vi "Find Average Center.vi"(5 "Position":i32, 7 "Tray Number":i32, 9 "XYZTheta":dbl[](array[numeric]), 10 "Motion.lvclass":refnum<class "Motion.lvclass">) -> (1 "XYZTheta":dbl[](array[numeric]), 2 "Motion Out":refnum<class "Motion.lvclass">)   [LabVIEW 2016, in "Component Tray.lvclass"]
uses:
  Component Tray.lvclass
  Find Component.ctl
  Controller/Motion/Motion.lvclass
  Controller/Camera/Machine Vision.ctl
  Controller/Camera/Edmund Optics/Edmund Optics.lvclass
  D:/UCSB-Gantry/V5/Classes/Controller/Camera/Camera.lvclass
  Controller/Camera/Camera.lvclass
panel:
  in  "Speed XY":dbl=5.0
  in  "Jog Cluster":T1={"Jog XY Cluster"={"object goes up"=FALSE, "object goes down"=FALSE, "object goes right"=FALSE, "object goes left"=FALSE, "SW2"=FALSE, "SW1"=FALSE, "YY (mm)"=0.1, "YN (mm) "=0.01, "NY (mm) "=0.005, "NN (mm) "=0.001}, "Jog Z Cluster "={"Z go down 0.1 mm"=FALSE, "Z go up 0.1 mm"=FALSE, "Z go down 0.05 mm"=FALSE, "Z go up 0.05 mm"=FALSE, "Z go down 0.01 mm"=FALSE, "Z go up 0.01 mm"=FALSE, "Z go down"=FALSE, "Z go up"=FALSE, "step (mm)"=0.001}}
  in  "Go 3":bool
  in  "light":dbl=5.0
  in  "Change light":bool
  out "Image 2":T2(plugin-control)
  in  "Machine Vision 2":T3
  in  "Machine Vision":T3
  out "Gantry":dbl[](array[numeric])
  out "Sum":dbl[](array[numeric])
  out "BR XY":dbl[](array[numeric])
  out "TR XY":dbl[](array[numeric])
  out "BL XY":dbl[](array[numeric])
  out "TL XY":dbl[](array[numeric])
  in  "Record Top Right":bool
  in  "Record Bottom Right":bool
  in  "Record Bottom Left":bool
  in  "Record Top Left":bool
  in  "Go to Bottom Right":bool
  in  "Go to Top Right":bool
  in  "Go to Bottom Left":bool
  in  "Go to Top Left":bool
  in  "Joystick":bool
  out "Camera":dbl[](array[numeric])
  in  "Go to Center":bool
  in  "Component":T4
  in  "Stop Program":bool
  out "Image":T2(plugin-control)
  # "1"
  # "2"
  # "Machine Vision:\nAcrylic : None"
  # "Light \nAcrylic : 5"
  # "--> Light on  : running\n       LIght off : Finish"
  # "Position 1"
  # "Position 2"
  # "Position 3"
  # "Position 4"
  # "Acrylic PCB"
  # "3"
  # "4"
  # "5"
  # "6"
  # "7"
  # "Component alignment 定位材料"
  # "8"
  # "9"
  # "10"
  # "11"
  # "12"
  # "1. Choose pattern recognition program 選擇視覺辨識\n2. Choose camera light luminosity 選擇亮度\n3. Go To Top Left  到第一定位點，點選Joystick進行定位\n4. Record Top Left 紀錄第一點\n5. Go To Bottom Left 到第二定位點，點選Joystick進行定位\n6. Record Bottom Left 紀錄第二點\n7. Go To Top Right 到第三定位點，點選Joystick進行定位\n8. Record Bottom Left 紀錄第二點\n9. Go To Bottom Left 到第四定位點，點選Joystick進行定位\n10. Record Bottom Left 紀錄第三點\n11. Go to Center 到中心點 檢查是否定位結果正常\n12. Submit 結束Component定位"
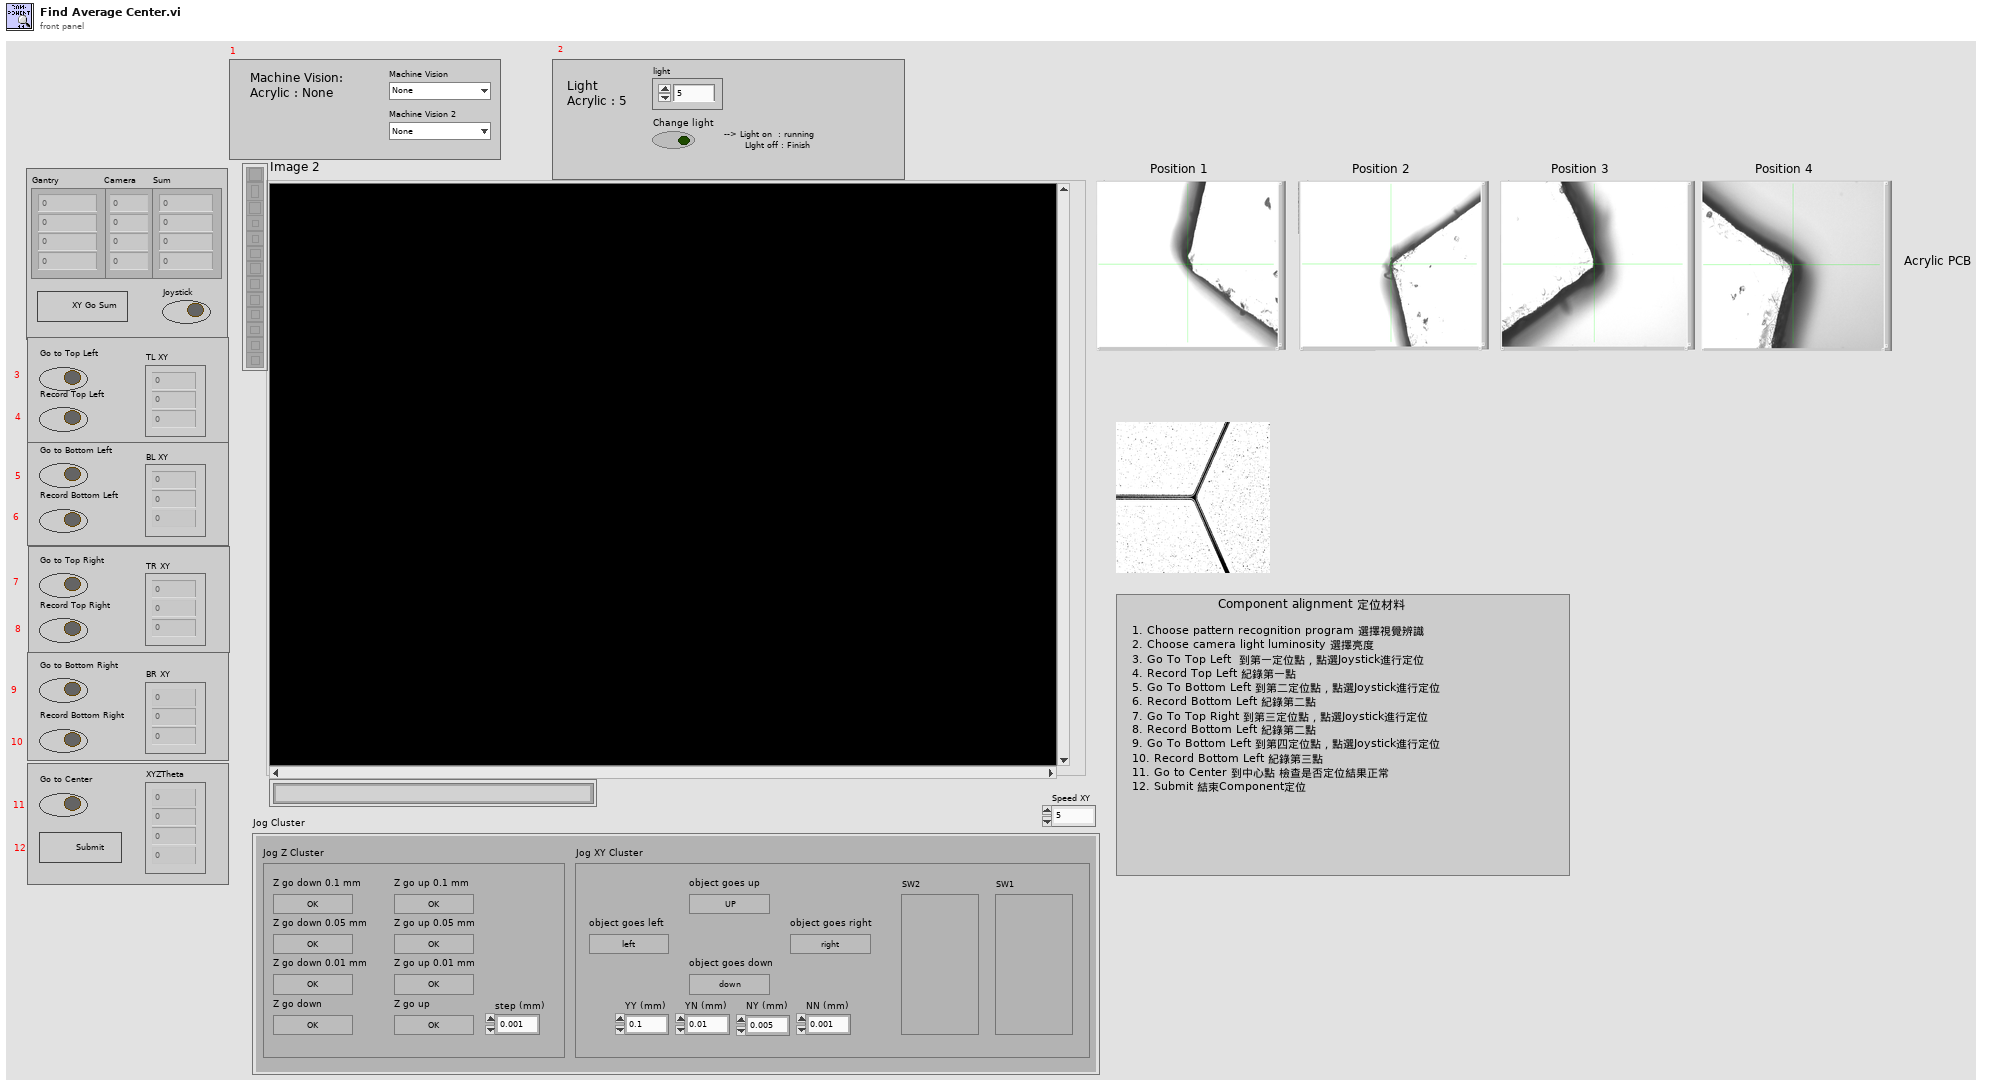
[diagram p1: front panel]
types:
  T1 = cluster{"Jog XY Cluster":cluster{"object goes up":bool, "object goes down":bool, "object goes right":bool, "object goes left":bool, "SW2":bool, "SW1":bool, "YY (mm)":dbl, "YN (mm) ":dbl, "NY (mm) ":dbl, "NN (mm) ":dbl}, "Jog Z Cluster ":cluster{"Z go down 0.1 mm":bool, "Z go up 0.1 mm":bool, "Z go down 0.05 mm":bool, "Z go up 0.05 mm":bool, "Z go down 0.01 mm":bool, "Z go up 0.01 mm":bool, "Z go down":bool, "Z go up":bool, "step (mm)":dbl}}
  T2 = typedef "IMAQ Image.ctl" = refnum<image>
  T3 = typedef "Camera.lvclass/Machine Vision.ctl" = enum16{"None", "Circle", "Tray Fiducials", "Tray Fiducials, top right", "HPK Silicon square", "HPK Silicon", "8inch PCB Pad", "Hexaboard", "Corner (TL, BR)", "Corner (BL, TR)"}
  T4 = typedef "Component Tray.lvclass/Find Component.ctl" = cluster{"New Fiducials":dbl[], "Past Fiducials":dbl[], "XYZTheta":dbl[], "Fiducials Path":path, "Position":i32}
  T5 = typedef "File Paths.ctl" = cluster{"Glue Pattern Folder":path, "Carrier Tray Folder":path, "Pick Up Tool Fixture Folder":path, "Components Folder":path, "Bellows Tool Offset.txt":path, "Pick Up Tool Offset.txt":path, "Dispense Tip Offset.txt":path, "Log Files":path}
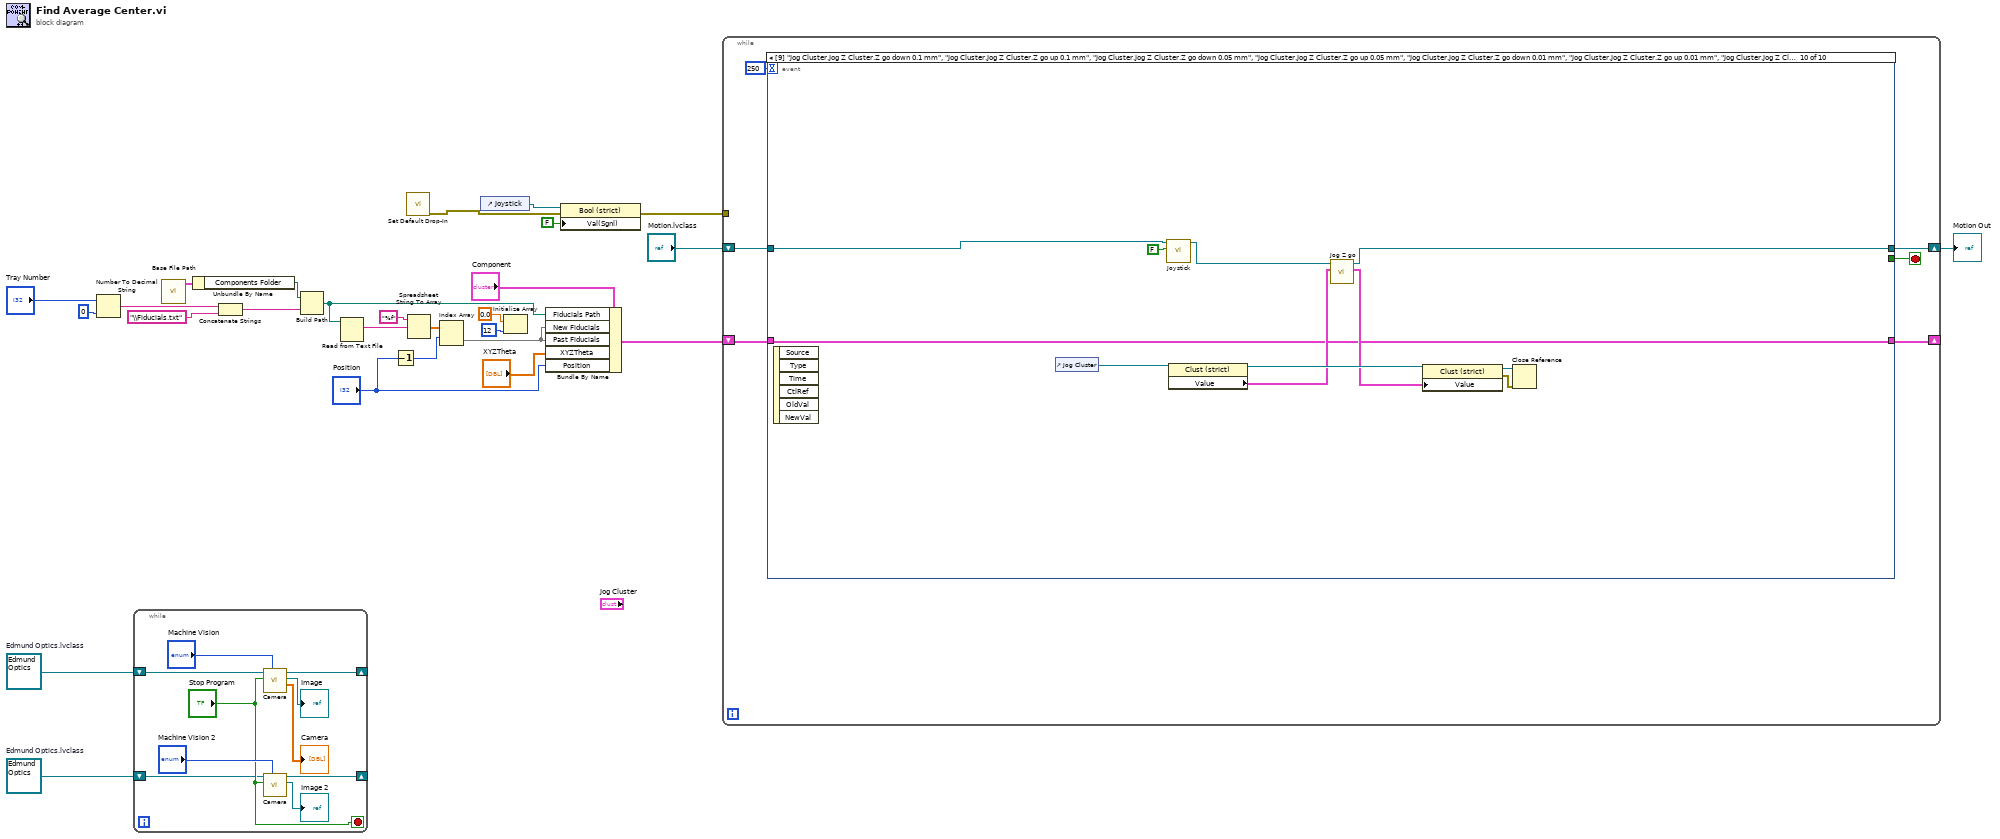
[diagram p0: block diagram]
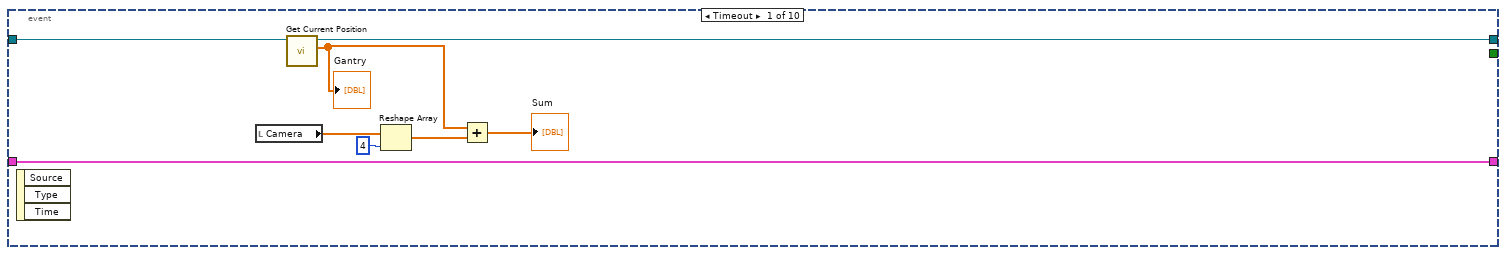
[diagram p2: hidden frame]
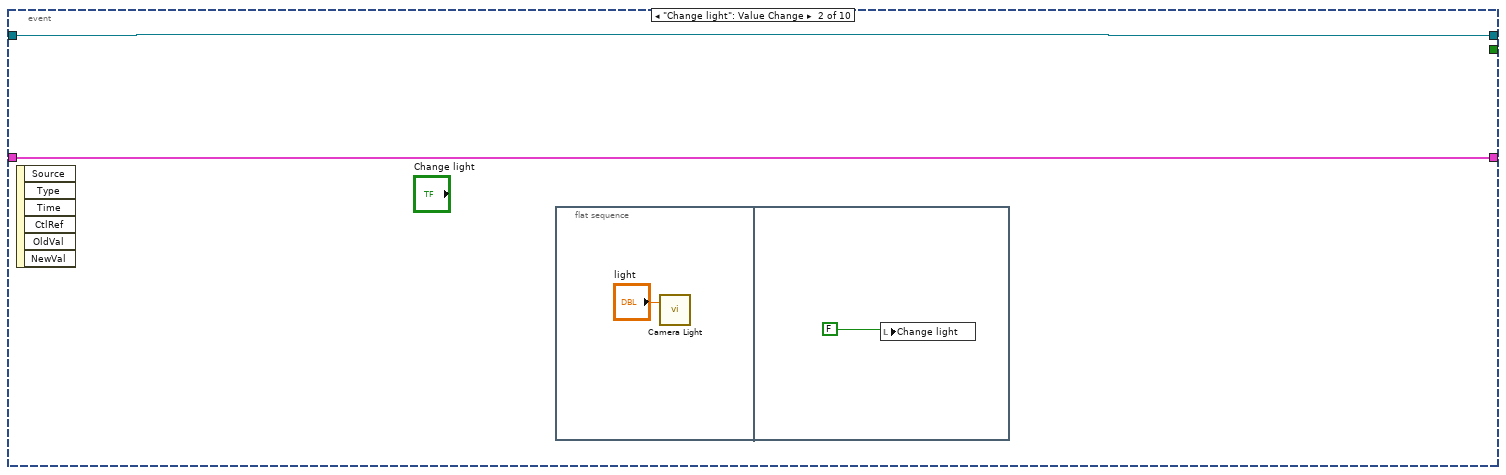
[diagram p3: hidden frame]
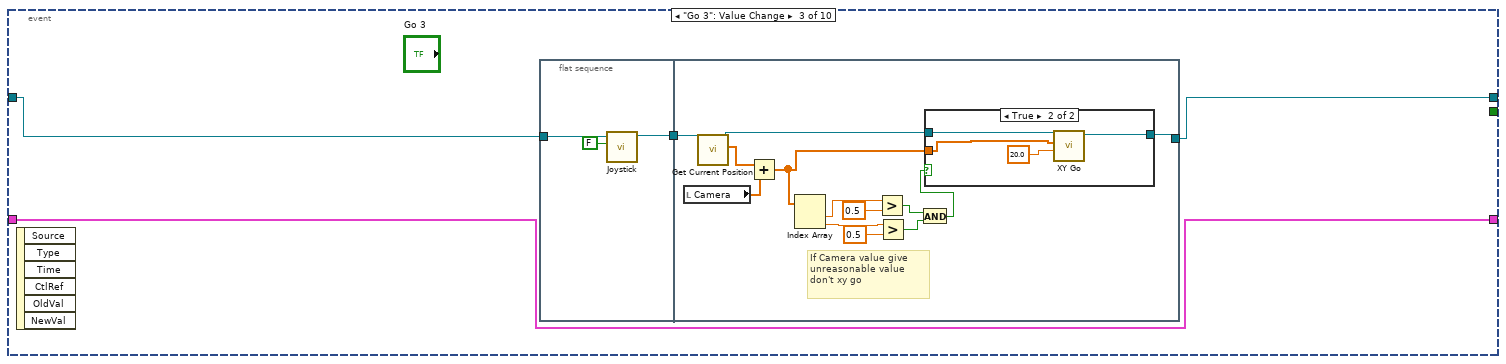
[diagram p4: hidden frame]
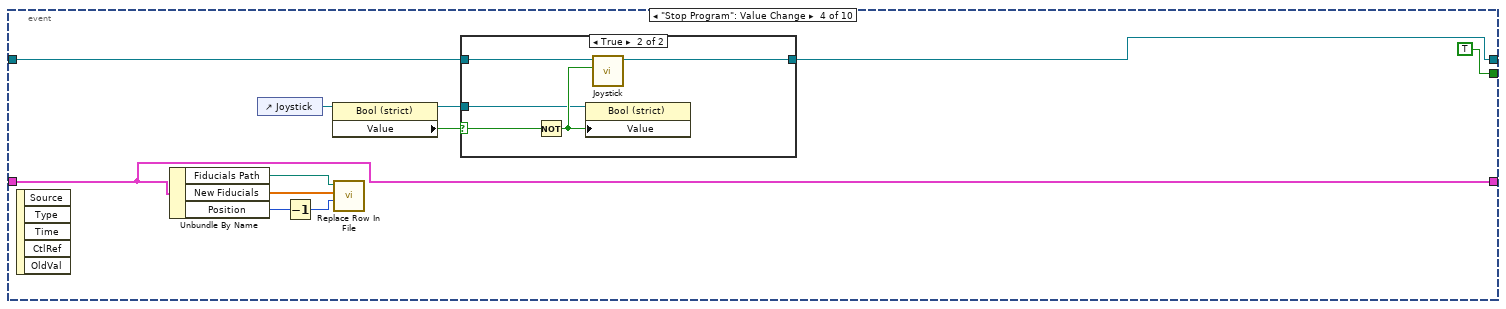
[diagram p6: hidden frame]
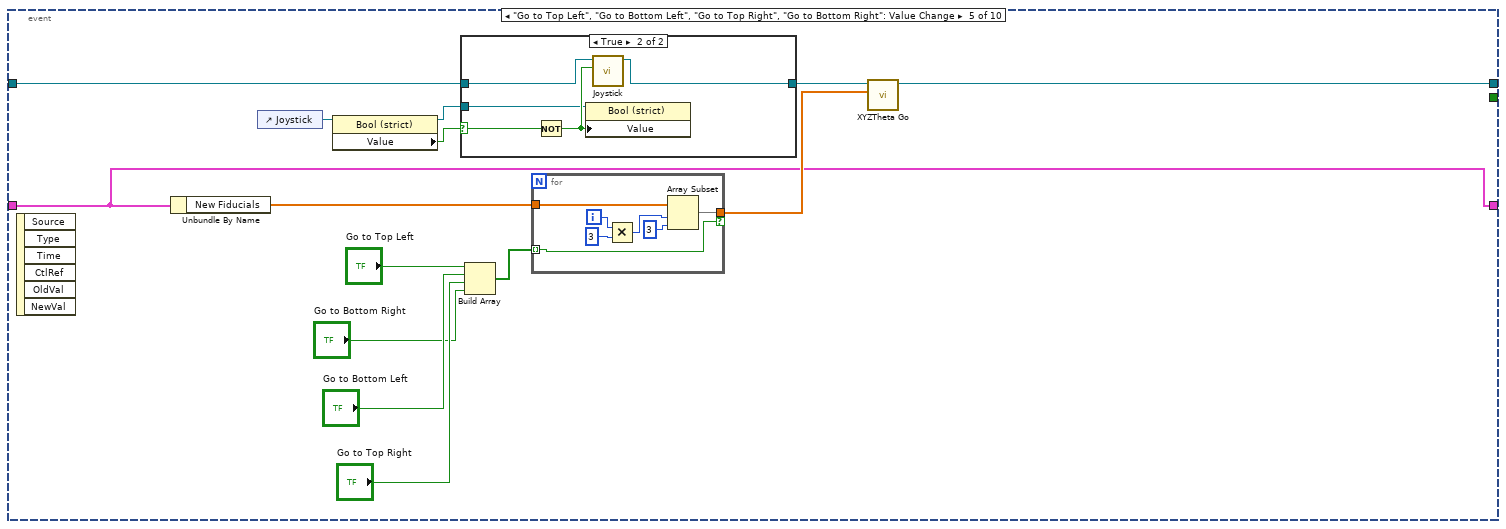
[diagram p8: hidden frame]
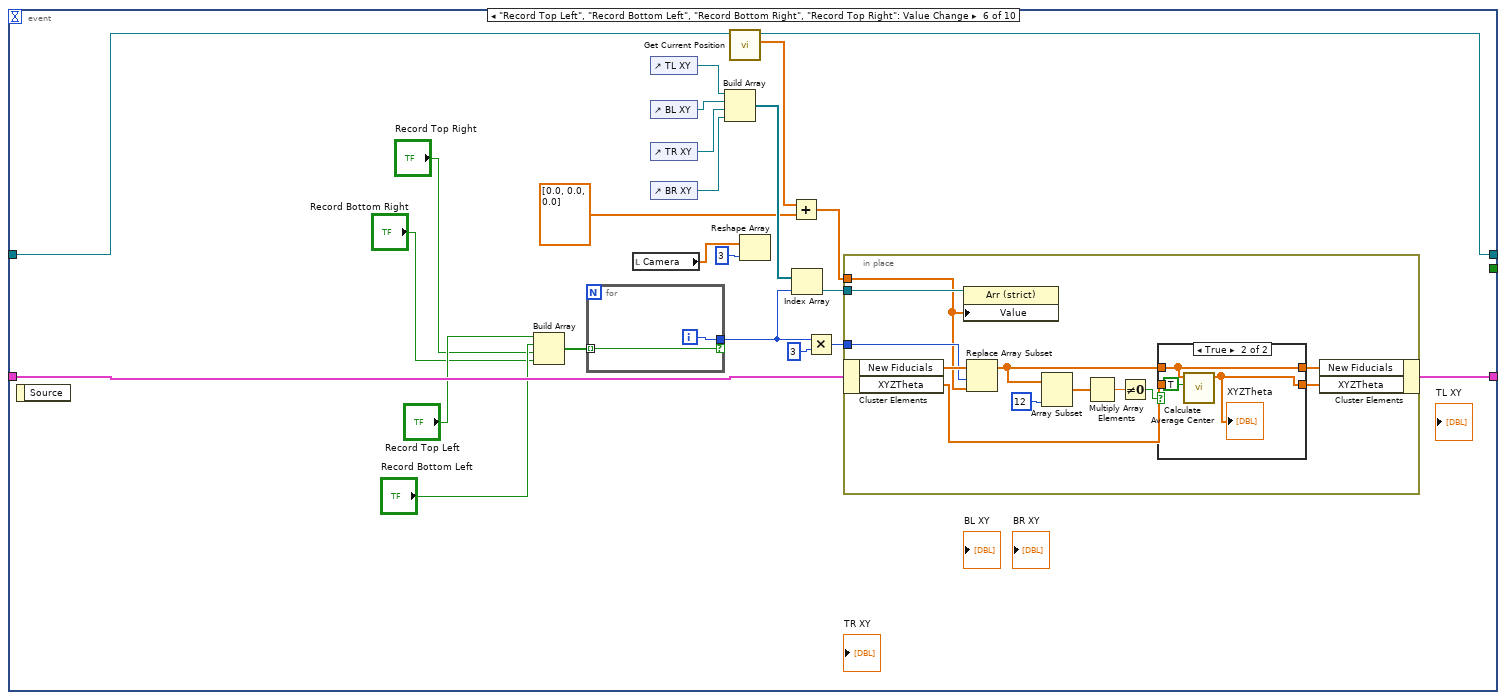
[diagram p10: hidden frame]
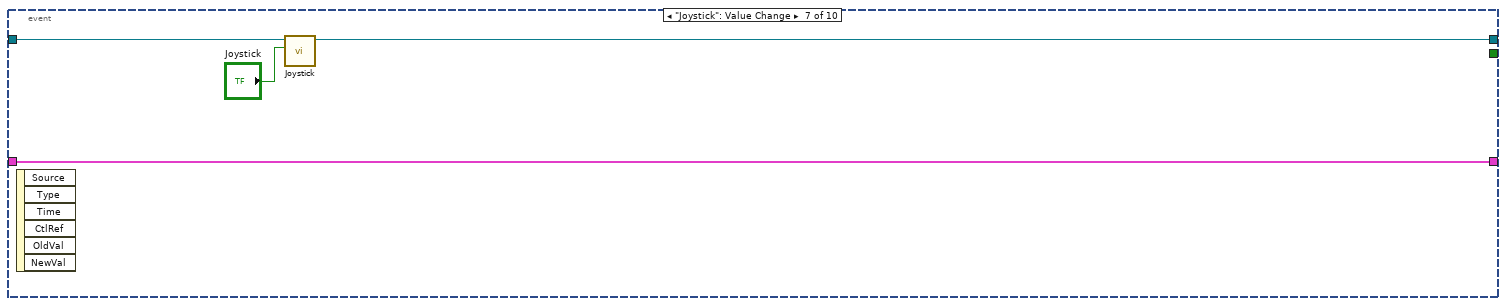
[diagram p12: hidden frame]
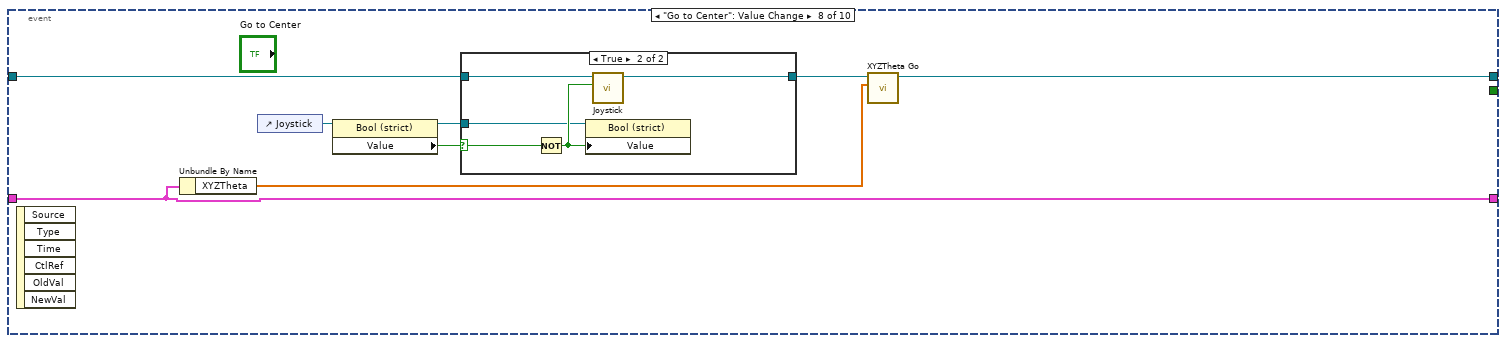
[diagram p13: hidden frame]
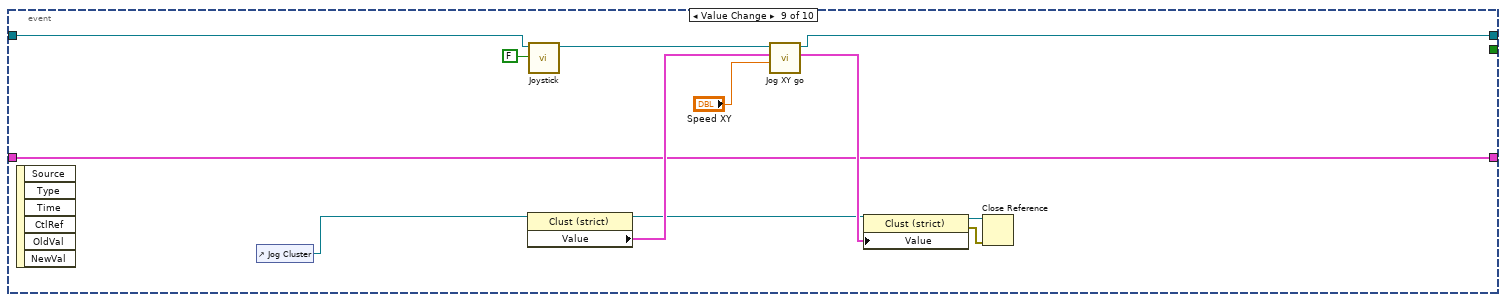
[diagram p15: hidden frame]
diagram:
  w2 = refnum<class "Edmund Optics.lvclass"> refnum  # Edmund Optics.lvclass
  w22 = refnum<class "Edmund Optics.lvclass"> refnum  # Edmund Optics.lvclass
  n1 = Number To Decimal String(number="Tray Number", width (-)=i16 0) -> (decimal integer string=w14:string)
  n2 = while {
    shift-right: [w33] -> _
    shift-left: w22 -> [w37]
    shift-right: [w29] -> _
    shift-left: w2 -> [w30]
    stop <- "Stop Program" stop-if-true
    n3 = call "Camera.vi"("Machine Vision"="Machine Vision", "Stop"="Stop Program", "Camera in"=w37) -> ("Camera"=→"Camera":dbl[], "Image"=→"Image":T2, "Camera out"=w33:refnum<class "Edmund Optics.lvclass">)  [unwired: 5 in, 1 out]
    n4 = call "Camera.vi"("Machine Vision"="Machine Vision 2", "Stop"="Stop Program", "Camera in"=w30) -> ("Image"=→"Image 2":T2, "Camera out"=w29:refnum<class "Edmund Optics.lvclass">)  [unwired: 5 in, 2 out]
  }
  n5 = call "Base File Path.vi"() -> ("Paths Out"=w11:T5)  [unwired: 11 in]
  n6 = Unbundle By Name(w11) -> ("Components Folder"=w13:path)
  n7 = Concatenate Strings(w14, "\\Fiducials.txt" ("string")) -> (w16:string)
  n8 = Build Path(base path=w13, name or relative path=w16) -> (appended path=w7:path)
  n9 = Read from Text File(file (use dialog)=w7) -> (text=w17:string)  [unwired: 3 in, 3 out]
  n10 = Decrement(x="Position") -> (x-1=w4:i32)
  n11 = call "Set Default Drop-In.vi"() -> ("error out"=w3:errorcluster)  [unwired: 11 in]
  n12 = Spreadsheet String To Array(format string="%f", spreadsheet string=w17) -> (array=w19:dbl[][])  [unwired: 2 in]
  n13 = Index Array(array=w19, index (row)=w4) -> (element=w1:dbl[])  [unwired: 1 in]
  n14 = control-ref of="Joystick"() -> (w25:refnum<vi>)
  n15 = Initialize Array(0.0 ("element"), 12 ("dimension size")) -> ()  [unwired: 1 out]
  n16 = Bundle By Name(cluster="Component", "Fiducials Path"=w7, "New Fiducials"=w1, "Past Fiducials"=w1, "XYZTheta"="XYZTheta", "Position"="Position") -> (w26:T4)
  n17 = property class="Bool (strict)"(reference=w25, error in=w3, "Val(Sgnl)"=FALSE) -> (error out=w23:errorcluster)  [unwired: 1 out]
  n18 = while {
    shift-right: [w41] -> _
    shift-left: w26 -> [w42]
    tunnel: w23 -> [_]
    shift-right: [w39] -> w20
    shift-left: "Motion.lvclass" -> [w38]
    stop <- w43 stop-if-true
    n19 = event shown="[9] \"Jog Cluster.Jog Z Cluster.Z go down 0.1 mm\", \"Jog Cluster.Jog Z Cluster.Z go up 0.1 mm\", \"Jog Cluster.Jog Z Cluster.Z go down 0.05 mm\", \"Jog Cluster.Jog Z Cluster.Z go up 0.05 mm\", \"Jog Cluster.Jog Z Cluster.Z go down 0.01 mm\", \"Jog Cluster.Jog Z Cluster.Z go up 0.01 mm\", \"Jog Cluster.Jog Z Cluster.Z go down\", \"Jog Cluster.Jog Z Cluster.Z go up\": Value Change" {
      selector: _ -> [_ _ _ _ _ _ _ _ _ _]
      dyn-events: _ -> [_ _ _ _ _ _ _ _ _ _]
      timeout: 250 -> [_ _ _ _ _ _ _ _ _ _]
      tunnel: [_ _ _ TRUE _ _ _ _ _ _] -> w43
      tunnel: w42 -> [w49 w52 w56 w85 w104 w147 w169 w176 w185 w197]
      tunnel: [w49 w52 w56 w85 w104 w146 w169 w176 w185 w197] -> w41
      tunnel: w38 -> [w50 w53 w58 w87 w100 w134 w168 w172 w188 w199]
      tunnel: [w48 w53 w57 w86 w103 w133 w167 w177 w186 w198] -> w39
      event Timeout {
        n20 = event-data() -> ()  [unwired: 1 in, 3 out]
        n21 = local read "Camera"() -> (w47:dbl[])
        n22 = call-dynamic "Get Current Position.vi"("Motion in"=w50) -> ("XYZTheta Out"=w51:dbl[], "Motion out"=w48:refnum<class "Motion.lvclass">)  [unwired: 8 in, 1 out]
        "Gantry" <- w51
        n23 = Reshape Array(w47, 4 ("dimension size")) -> (w45:dbl[])
        n24 = Add(x=w51, y=w45) -> (x+y=→"Sum":dbl[])
      }
      event "Change light": Value Change {
        n25 = event-data() -> ()  [unwired: 1 in, 6 out]
        n26 = flat-sequence {
          frame #0 {
            n27 = call "Camera Light.vi"("input"="light") -> ()  [unwired: 2 in, 1 out]
          }
          frame #1 {
            n28 = local write "Change light"(FALSE) -> ()
          }
        }
      }
      event "Go 3": Value Change {
        n29 = event-data() -> ()  [unwired: 1 in, 6 out]
        n30 = flat-sequence {
          tunnel: w58 -> [w62]
          tunnel: [w60] -> w59
          tunnel: w59 -> [w68]
          tunnel: [w75] -> w57
          frame #0 {
            n31 = call-dynamic "Joystick.vi"("Joystick"=FALSE, "Motion in"=w62) -> ("Motion out"=w60:refnum<class "Motion.lvclass">)  [unwired: 8 in, 1 out]
          }
          frame #1 {
            # "If Camera value give unreasonable value \ndon't xy go"
            n32 = local read "Camera"() -> (w63:dbl[])
            n33 = call-dynamic "Get Current Position.vi"("Motion in"=w68) -> ("XYZTheta Out"=w66:dbl[], "Motion out"=w67:refnum<class "Motion.lvclass">)  [unwired: 8 in, 1 out]
            n34 = Add(x=w66, y=w63) -> (x+y=w65:dbl[])
            n35 = Index Array(array=w65) -> (element #1=w74:dbl, element #2=w72:dbl)  [unwired: 2 in]
            n36 = Greater?(x=w74, y=0.5) -> (0:w70:bool)
            n37 = Greater?(x=w72, y=0.5) -> (0:w69:bool)
            n38 = And(x=w70, y=w69) -> (x .and. y?=w64:bool)
            n39 = case shown="True" w64 {
              tunnel: w67 -> [w76 w80]
              tunnel: [w76 w79] -> w75
              tunnel: w65 -> [_ w77]
              frame False {
              }
              frame True {
                n40 = call-dynamic "XY Go.vi"("Speed"=20.0, "XY"=w77, "Motion in"=w80) -> ("Motion out"=w79:refnum<class "Motion.lvclass">)  [unwired: 7 in, 1 out]
              }
            }
          }
        }
      }
      event "Stop Program": Value Change {
        n41 = event-data() -> ()  [unwired: 1 in, 5 out]
        n42 = Unbundle By Name(w85) -> ("Fiducials Path"=w83:path, "New Fiducials"=w84:dbl[], "Position"=w82:i32)
        n43 = control-ref of="Joystick"() -> (w88:refnum<vi>)
        n44 = Decrement(x=w82) -> (x-1=w81:i32)
        n45 = property class="Bool (strict)"(reference=w88) -> (reference out=w89:refnum<vi>, "Value"=w90:bool)  [unwired: 1 in, 1 out]
        n46 = call "Replace Row In File.vi"("Index"=w81, "Insert Array"=w84, "Path"=w83) -> ()  [unwired: 8 in, 1 out]
        n47 = case shown="True" w90 {
          selector: w90 -> [_ w97]
          tunnel: w87 -> [w92 w96]
          tunnel: [w92 w95] -> w86
          tunnel: w89 -> [_ w93]
          frame False {
          }
          frame True {
            n48 = Not(x=w97) -> (.not. x?=w94:bool)
            n49 = property class="Bool (strict)"(reference=w93, "Value"=w94) -> ()  [unwired: 1 in, 2 out]
            n50 = call-dynamic "Joystick.vi"("Joystick"=w94, "Motion in"=w96) -> ("Motion out"=w95:refnum<class "Motion.lvclass">)  [unwired: 8 in, 1 out]
          }
        }
      }
      event "Go to Top Left", "Go to Bottom Left", "Go to Top Right", "Go to Bottom Right": Value Change {
        n51 = event-data() -> ()  [unwired: 1 in, 6 out]
        n52 = Unbundle By Name(w104) -> ("New Fiducials"=w106:dbl[])
        n53 = control-ref of="Joystick"() -> (w98:refnum<vi>)
        n54 = property class="Bool (strict)"(reference=w98) -> (reference out=w101:refnum<vi>, "Value"=w102:bool)  [unwired: 1 in, 1 out]
        n55 = case shown="True" w102 {
          selector: w102 -> [_ w117]
          tunnel: w100 -> [w112 w116]
          tunnel: [w112 w115] -> w99
          tunnel: w101 -> [_ w113]
          frame False {
          }
          frame True {
            n56 = Not(x=w117) -> (.not. x?=w114:bool)
            n57 = property class="Bool (strict)"(reference=w113, "Value"=w114) -> ()  [unwired: 1 in, 2 out]
            n58 = call-dynamic "Joystick.vi"("Joystick"=w114, "Motion in"=w116) -> ("Motion out"=w115:refnum<class "Motion.lvclass">)  [unwired: 8 in, 1 out]
          }
        }
        n59 = Build Array("Go to Top Left", "Go to Bottom Left", "Go to Top Right", "Go to Bottom Right") -> (w107:bool[])
        n60 = for {
          tunnel: w107 -> [w124] mode=indexing
          tunnel: w106 -> [w123]
          tunnel: [w118] -> w105 if=w124
          i -> [w121]
          n61 = Multiply(x=w121, y=3) -> (x*y=w119:i32)
          n62 = Array Subset(array=w123, index=w119, length=3) -> (w118:dbl[])
        }
        n63 = call "XYZTheta Go.vi"("XYZTheta In"=w105, "Motion in"=w99) -> ("Motion out"=w103:refnum<class "Motion.lvclass">)  [unwired: 7 in, 2 out]
      }
      event "Record Top Left", "Record Bottom Left", "Record Bottom Right", "Record Top Right": Value Change {
        n64 = event-data() -> ()  [unwired: 1 in, 1 out]
        n65 = Build Array("Record Top Left", "Record Bottom Left", "Record Top Right", "Record Bottom Right") -> (w141:bool[])
        n66 = for {
          tunnel: w141 -> [w148] mode=indexing
          tunnel: [w149] -> w130 if=w148
          i -> [w149]
        }
        n67 = local read "Camera"() -> (w127:dbl[])
        n68 = control-ref of="TL XY"() -> (w140:refnum<vi>)
        n69 = control-ref of="BL XY"() -> (w139:refnum<vi>)
        n70 = control-ref of="TR XY"() -> (w138:refnum<vi>)
        n71 = control-ref of="BR XY"() -> (w137:refnum<vi>)
        n72 = Build Array(w140, w139, w138, w137) -> (w136:refnum<vi>[])
        n73 = call-dynamic "Get Current Position.vi"("Motion in"=w134) -> ("XYZTheta Out"=w132:dbl[], "Motion out"=w133:refnum<class "Motion.lvclass">)  [unwired: 8 in, 1 out]
        n74 = Reshape Array(w127, 3 ("dimension size")) -> ()  [unwired: 1 out]
        n75 = Add(x=w132, y=dbl[] [0.0, 0.0, 0.0]) -> (x+y=w126:dbl[])
        n76 = Index Array(array=w136, index=w130) -> (element=w135:refnum<vi>)
        n77 = Multiply(x=w130, y=3) -> (x*y=w128:i32)
        n78 = in-place {
          in-place-border: w128 -> [w159]
          in-place-border: w135 -> [w156]
          in-place-border: w126 -> [w154]
          n79 = in-place-cluster #1(w147) -> ("New Fiducials"=w160:dbl[], "XYZTheta"=w155:dbl[])
          n80 = property class="Arr (strict)"(reference=w156, "Value"=w154) -> ()  [unwired: 1 in, 2 out]
          n81 = Replace Array Subset(array=w160, new element=w154, index=w159) -> (w153:dbl[])
          n82 = Array Subset(array=w153, length=12) -> (w151:dbl[])  [unwired: 1 in]
          n83 = Multiply Array Elements(1:w151) -> (0:w150:dbl)
          n84 = Not Equal To 0?(x=w150) -> (x != 0?=w157:bool)
          n85 = case shown="True" w157 {
            tunnel: [w162 w165] -> w161
            tunnel: w153 -> [w163 w166]
            tunnel: [w163 w166] -> w158
            tunnel: w155 -> [w162 _]
            frame False {
            }
            frame True {
              n86 = call "Calculate Average Center.vi"("Boolean"=TRUE, "Gantry Fiducials"=w166) -> ("XYZTheta"=w165:dbl[])  [unwired: 9 in]
              "XYZTheta" <- w165
            }
          }
          n87 = in-place-cluster #1("New Fiducials"=w158, "XYZTheta"=w161) -> (w146:T4)
        }
      }
      event "Joystick": Value Change {
        n88 = event-data() -> ()  [unwired: 1 in, 6 out]
        n89 = call-dynamic "Joystick.vi"("Joystick"="Joystick", "Motion in"=w168) -> ("Motion out"=w167:refnum<class "Motion.lvclass">)  [unwired: 8 in, 1 out]
      }
      event "Go to Center": Value Change {
        n90 = event-data() -> ()  [unwired: 1 in, 6 out]
        n91 = Unbundle By Name(w176) -> ("XYZTheta"=w178:dbl[])
        n92 = control-ref of="Joystick"() -> (w173:refnum<vi>)
        n93 = property class="Bool (strict)"(reference=w173) -> (reference out=w174:refnum<vi>, "Value"=w175:bool)  [unwired: 1 in, 1 out]
        n94 = case shown="True" w175 {
          selector: w175 -> [_ w184]
          tunnel: w172 -> [w179 w183]
          tunnel: [w179 w182] -> w171
          tunnel: w174 -> [_ w180]
          frame False {
          }
          frame True {
            n95 = Not(x=w184) -> (.not. x?=w181:bool)
            n96 = property class="Bool (strict)"(reference=w180, "Value"=w181) -> ()  [unwired: 1 in, 2 out]
            n97 = call-dynamic "Joystick.vi"("Joystick"=w181, "Motion in"=w183) -> ("Motion out"=w182:refnum<class "Motion.lvclass">)  [unwired: 8 in, 1 out]
          }
        }
        n98 = call "XYZTheta Go.vi"("XYZTheta In"=w178, "Motion in"=w171) -> ("Motion out"=w177:refnum<class "Motion.lvclass">)  [unwired: 7 in, 2 out]
      }
      event "Jog Cluster.Jog XY Cluster.object goes up", "Jog Cluster.Jog XY Cluster.object goes down", "Jog Cluster.Jog XY Cluster.object goes right", "Jog Cluster.Jog XY Cluster.object goes left": Value Change {
        n99 = event-data() -> ()  [unwired: 1 in, 6 out]
        n100 = control-ref of="Jog Cluster"() -> (w187:refnum<vi>)
        n101 = property class="Clust (strict)"(reference=w187) -> (reference out=w192:refnum<vi>, "Value"=w194:T1)  [unwired: 1 in, 1 out]
        n102 = call-dynamic "Joystick.vi"("Joystick"=FALSE, "Motion in"=w188) -> ("Motion out"=w189:refnum<class "Motion.lvclass">)  [unwired: 8 in, 1 out]
        n103 = call "Jog XY go.vi"("Speed"="Speed XY", "Jog Cluster IN"=w194, "Motion.lvclass IN"=w189) -> ("Jog Cluster OUT"=w193:T1, "Motion.lvclass OUT"=w186:refnum<class "Motion.lvclass">)  [unwired: 7 in]
        n104 = property class="Clust (strict)"(reference=w192, "Value"=w193) -> (reference out=w190:refnum<vi>, error out=w191:errorcluster)  [unwired: 1 in]
        n105 = Close Reference(reference=w190, error in (no error)=w191) -> ()  [unwired: 1 out]
      }
      event "Jog Cluster.Jog Z Cluster.Z go down 0.1 mm", "Jog Cluster.Jog Z Cluster.Z go up 0.1 mm", "Jog Cluster.Jog Z Cluster.Z go down 0.05 mm", "Jog Cluster.Jog Z Cluster.Z go up 0.05 mm", "Jog Cluster.Jog Z Cluster.Z go down 0.01 mm", "Jog Cluster.Jog Z Cluster.Z go up 0.01 mm", "Jog Cluster.Jog Z Cluster.Z go down", "Jog Cluster.Jog Z Cluster.Z go up": Value Change {
        n106 = event-data() -> ()  [unwired: 1 in, 6 out]
        n107 = control-ref of="Jog Cluster"() -> (w200:refnum<vi>)
        n108 = call-dynamic "Joystick.vi"("Joystick"=FALSE, "Motion in"=w199) -> ("Motion out"=w201:refnum<class "Motion.lvclass">)  [unwired: 8 in, 1 out]
        n109 = property class="Clust (strict)"(reference=w200) -> (reference out=w207:refnum<vi>, "Value"=w204:T1)  [unwired: 1 in, 1 out]
        n110 = call "Jog Z go.vi"("Jog Cluster IN"=w204, "Motion.lvclass IN"=w201) -> ("Jog Cluster OUT"=w203:T1, "Motion.lvclass OUT"=w198:refnum<class "Motion.lvclass">)  [unwired: 8 in]
        n111 = property class="Clust (strict)"(reference=w207, "Value"=w203) -> (reference out=w205:refnum<vi>, error out=w206:errorcluster)  [unwired: 1 in]
        n112 = Close Reference(reference=w205, error in (no error)=w206) -> ()  [unwired: 1 out]
      }
    }
  }
  "Motion Out" <- w20
